vi "Generic Dialog.vi"(10 "message Input":string="<b>--WARNING---</b>\\nThis Module's path is \\n\\n<b><%s></b>\\n\\n If you continue, you will probably be modifying a dependency or a VIP Package, do you want to proceed?") -> (3 "Continue?":bool)   [LabVIEW 2020, in "Panther Dashboard.lvlib"]
uses:
  Panther Dashboard.lvlib
  Controls/Continue.ctl
panel:
  in  "Continue":T1
  out "Message":string
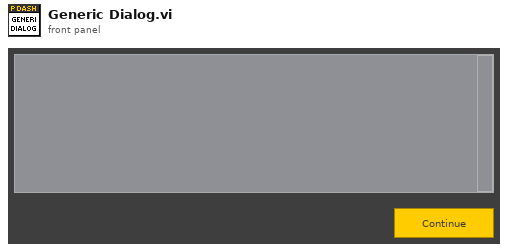
[diagram p1: front panel]
types:
  T1 = typedef "Continue.ctl" = bool
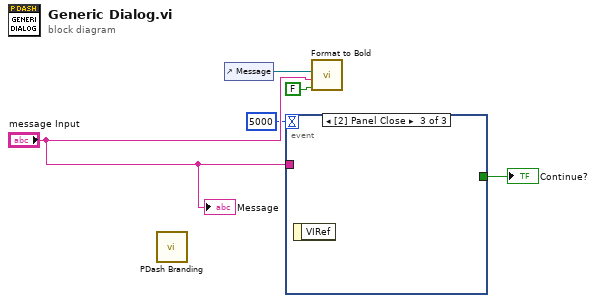
[diagram p0: block diagram]
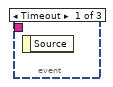
[diagram p2: hidden frame]
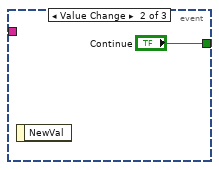
[diagram p3: hidden frame]
diagram:
  n1 = call "PDash Branding.vi"() -> ()  [unwired: 12 in]
  n2 = control-ref of="Message"() -> (w5:refnum<vi>)
  n3 = event shown="[2] Panel Close" {
    selector: _ -> [_ _ _]
    dyn-events: _ -> [_ _ _]
    timeout: 5000 -> [_ _ _]
    tunnel: [_ "Continue" _] -> w3
    tunnel: "message Input" -> [_ _ _]
    event Timeout {
      n4 = event-data() -> ()  [unwired: 1 in, 1 out]
    }
    event Value Change {
      n5 = event-data() -> ()  [unwired: 1 in, 1 out]
    }
    event Panel Close {
      n6 = event-data() -> ()  [unwired: 1 in, 1 out]
    }
  }
  "Continue?" <- w3
  n7 = call "Format to Bold.vi"("Adjust Height?"=FALSE, "String Value"="message Input", "String Ref"=w5) -> ()  [unwired: 9 in]
  "Message" <- "message Input"
